vi "Call Refprop.vi"(0 "fluid name":u16(ring)=17 items=["AIR.MIX", "AMARILLO.MIX", "EKOFISK.MIX", "GLFCOAST.MIX", "HIGHCO2.MIX", "HIGHN2.MIX", "NGSAMPLE.MIX", "R401A.MIX", "R401B.MIX", "R401C.MIX", "R402A.MIX", "R402B.MIX", "R403A.MIX", "R403B.MIX", "R405A.MIX", "R406A.MIX", "R407A.MIX", "R407B.MIX", "R407C.MIX", "R407D.MIX", "R407E.MIX", "R408A.MIX", "R409A.MIX", "R409B.MIX", "R410A.PPF", "R410B.MIX", "R411A.MIX", "R411B.MIX", "R412A.MIX", "R413A.MIX", "R414B.MIX", "R415A.MIX", "R415B.MIX", "R416A.MIX", "R417A.MIX", "R417B.MIX", "R417C.MIX", "R418A.MIX", "R419A.MIX", "R419B.MIX", "R420A.MIX", "R421A.MIX", "R421B.MIX", "R422A.MIX", "R422B.MIX", "R422C.MIX", "R422D.MIX", "R423A.MIX", "R424A.MIX", "R425A.MIX", "R426A.MIX", "R427A.MIX", "R428A.MIX", "R429A.MIX", "R430A.MIX", "R431A.MIX", "R432A.MIX", "R433A.MIX", "R433B.MIX", "R433C.MIX", "R434A.MIX", "R435A.MIX", "R436A.MIX", "R436B.MIX", "R437A.MIX", "R438A.MIX", "R439A.MIX", "R440A.MIX", "R441A.MIX", "R442A.MIX", "R443A.MIX", "R444A.MIX", "R444B.MIX", "R445A.MIX", "R446A.MIX", "R447A.MIX", "R448A.MIX", "R449A.MIX", "R449B.MIX", "R450A.MIX", "R451A.MIX", "R451B.MIX", "R452A.MIX", "R452B.MIX", "R452C.MIX", "R453A.MIX", "R454A.MIX", "R454B.MIX", "R454C.MIX", "R455A.MIX", "R456A.MIX", "R457A.MIX", "R459A.MIX", "R459B.MIX", "R460A.MIX", "R460B.MIX", "R500.MIX", "R501.MIX", "R502.MIX", "R503.MIX", "R504.MIX", "R507A.MIX", "R508A.MIX", "R508B.MIX", "R509A.MIX", "R510A.MIX", "R511A.MIX", "R512A.MIX", "R513A.MIX", "R513B.MIX", "R515A.MIX", "ammonia.fld", "butane.fld", "ethane.fld", "propane.fld", "R11.fld", "R113.fld", "R114.fld", "R115.fld", "R116.fld", "R12.fld", "R123.fld", "R124.fld", "R125.fld", "R13.fld", "R134a.fld", "R14.fld", "R141b.fld", "R142b.fld", "R143a.fld", "R152a.fld", "R161.fld", "R21.fld", "R218.fld", "R22.fld", "R227ea.fld", "R23.fld", "R236ea.fld", "R236fa.fld", "R245ca.fld", "R245fa.fld", "R32.fld", "R41.fld", "R1216.fld", "RC318.fld", "water.fld", "1butene.fld", "acetone.fld", "argon.fld", "benzene.fld", "c1cc6.fld", "c2butene.fld", "c3cc6.fld", "c4f10.fld", "c5f12.fld", "c11.fld", "c12.fld", "cf3i.fld", "CO.fld", "CO2.fld", "COS.fld", "cyclohex.fld", "cyclopen.fld", "cyclopro.fld", "D2.fld", "D2O.fld", "D4.fld", "D5.fld", "D6.fld", "decane.fld", "dee.fld", "dmc.fld", "dme.fld", "ebenzene.fld", "ethanol.fld", "ethylene.fld", "flourine.fld", "H2S.fld", "HCl.fld", "helium.fld", "heptane.fld", "hexane.fld", "hydrogen.fld", "ibutene.fld", "ihexane.fld", "ioctane.fld", "ipentane.fld", "isobutan.fld", "krypton.fld", "MD2M.fld", "MD3M.fld", "MD4M.fld", "MDM.fld", "methane.fld", "methanol.fld", "mlinolea.fld", "mlinolen.fld", "MM.fld", "moleate.fld", "mpalmita.fld", "mstearat.fld", "mxylene.fld", "N2O.fld", "neon.fld", "neopentn.fld", "NF3.fld", "nitrogen.fld", "nonane.fld", "novec649.fld", "octane.fld", "orthohyd.fld", "oxygen.fld", "parahyd.fld", "pentane.fld", "propylen.fld", "propyne.fld", "pxylene.fld", "R365MFC.fld", "R1233zd.fld", "R1234yf.fld", "R1234ze.fld", "RE143a.fld", "RE245cb2.fld", "RE245fa2.fld", "RE347mcc.fld", "sf6.fld", "SO2.fld", "T2butene.fld", "xenon.fld"], 1 "units":enum16{"SI", "IP"}(ring), 5 "InpCode":T1(ring)=enum."TP", 9 "output_1":dbl=40.0, 11 "output_2":dbl=632.0) -> (4 "data":string[][](table)=[["0", "T", "40.917420"], ["1", "P", "632.917420"], ["2", "H", "466.332574"], ["3", "S", "2.054657"], ["4", "DV", "18.926081"], ["5", "DL", "18.926081"], ["6", "E", "432.891028"], ["7", "CV", "0.758226"], ["8", "CP", "0.924261"], ["9", "W", "194.299169"], ["10", "Q", "998.000000"]], 6 "Component Molar Fractions":dbl[](array[numeric]), 8 "Critical temperature (K)":dbl, 10 "Molecular Weight":dbl=72.58534253397343 format="%#_11g", 15 "Critical Pressure (kPa)":dbl)   [LabVIEW 2017]
panel:
  out "Components":i32=2
  out "refprop_main_directory":string="D:\\ni files\\refproplv\\cll_refprop_dll_on_lv"
  out "xmlout":string="<Array>\r\n<Name></Name>\r\n<Dimsize>39</Dimsize>\r\n<Dimsize>2</Dimsize>\r\n<String>\r\n<Name>String</Name>\r\n<Val>ammonia</Val>\r\n</String>\r\n<String>\r\n<Name>String</Name>\r\n<Val>ammonia</Val>\r\n</String>\r\n<String>\r\n<Name>String</Name>\r\n<Val>argon</Val>\r\n</String>\r\n<String>\r\n<Name>String</Name>\r\n<Val>argon</Val>\r\n</String>\r\n<String>\r\n<Name>String</Name>\r\n<Val>butane</Val>\r\n</String>\r\n<String>\r\n<Name>String</Name>\r\n<Val>n-butane</Val>\r\n</String>\r\n<String>\r\n<Name>String</Name>\r\n<Val>carbon dioxide</Val>\r\n</String>\r\n<String>\r\n<Name>String</Name>\r\n<Val>carbon dioxide</Val>\r\n</String>\r\n<String>\r\n<Name>String</Name>\r\n<Val>ethane</Val>\r\n</String>\r\n<String>\r\n<Name>String</Name>\r\n<Val>ethane</Val>\r\n</String>\r\n<String>\r\n<Name>String</Name>\r\n<Val>isobutane</Val>\r\n</String>\r\n<String>\r\n<Name>String</Name>\r\n<Val>2-methylpropane</Val>\r\n</String>\r\n<String>\r\n<Name>String</Name>\r\n<Val>methane</Val>\r\n</String>\r\n<String>\r\n<Name>String</Name>\r\n<Val>methane</Val>\r\n</String>\r\n<String>\r\n<Name>String</Name>\r\n<Val>nitrogen</Val>\r\n</String>\r\n<String>\r\n<Name>String</Name>\r\n<Val>nitrogen</Val>\r\n</String>\r\n<String>\r\n<Name>String</Name>\r\n<Val>oxygen</Val>\r\n</String>\r\n<String>\r\n<Name>String</Name>\r\n<Val>oxygen</Val>\r\n</String>\r\n<String>\r\n<Name>String</Name>\r\n<Val>propane</Val>\r\n</String>\r\n<String>\r\n<Name>String</Name>\r\n<Val>propane</Val>\r\n</String>\r\n<String>\r\n<Name>String</Name>\r\n<Val>propylene</Val>\r\n</String>\r\n<String>\r\n<Name>String</Name>\r\n<Val>propene</Val>\r\n</String>\r\n<String>\r\n<Name>String</Name>\r\n<Val>R11</Val>\r\n</String>\r\n<String>\r\n<Name>String</Name>\r\n<Val>trichlorofluoromethane</Val>\r\n</String>\r\n<String>\r\n<Name>String</Name>\r\n<Val>R113</Val>\r\n</String>\r\n<String>\r\n<Name>String</Name>\r\n<Val>1,1,2-trichloro-1,2,2-trifluoroethane</Val>\r\n</String>\r\n<String>\r\n<Name>String</Name>\r\n<Val>R114</Val>\r\n</String>\r\n<String>\r\n<Name>String</Name>\r\n<Val>1,2-dichloro-1,1,2,2-tetrafluoroethane</Val>\r\n</String>\r\n<String>\r\n<Name>String</Name>\r\n<Val>R115</Val>\r\n</String>\r\n<String>\r\n<Name>String</Name>\r\n<Val>chloropentafluoroethane</Val>\r\n</String>\r\n<String>\r\n<Name>String</Name>\r\n<Val>R116</Val>\r\n</String>\r\n<String>\r\n<Name>String</Name>\r\n<Val>hexafluoroethane</Val>\r\n</String>\r\n<String>\r\n<Name>String</Name>\r\n<Val>R12</Val>\r\n</String>\r\n<String>\r\n<Name>String</Name>\r\n<Val>dichlorodifluoromethane</Val>\r\n</String>\r\n<String>\r\n<Name>String</Name>\r\n<Val>R123</Val>\r\n</String>\r\n<String>\r\n<Name>String</Name>\r\n<Val>2,2-dichloro-1,1,1-trifluoroethane</Val>\r\n</String>\r\n<String>\r\n<Name>String</Name>\r\n<Val>R124</Val>\r\n</String>\r\n<String>\r\n<Name>String</Name>\r\n<Val>1-chloro-1,2,2,2-tetrafluoroethane</Val>\r\n</String>\r\n<String>\r\n<Name>String</Name>\r\n<Val>R125</Val>\r\n</String>\r\n<String>\r\n<Name>String</Name>\r\n<Val>pentafluoroethane</Val>\r\n</String>\r\n<String>\r\n<Name>String</Name>\r\n<Val>R13</Val>\r\n</String>\r\n<String>\r\n<Name>String</Name>\r\n<Val>chlorotrifluoromethane</Val>\r\n</String>\r\n<String>\r\n<Name>String</Name>\r\n<Val>R134a</Val>\r\n</String>\r\n<String>\r\n<Name>String</Name>\r\n<Val>1,1,1,2-tetrafluoroethane</Val>\r\n</String>\r\n<String>\r\n<Name>String</Name>\r\n<Val>R14</Val>\r\n</String>\r\n<String>\r\n<Name>String</Name>\r\n<Val>tetrafluoromethane</Val>\r\n</String>\r\n<String>\r\n<Name>String</Name>\r\n<Val>R141b</Val>\r\n</String>\r\n<String>\r\n<Name>String</Name>\r\n<Val>1,1-dichloro-1-fluoroethane</Val>\r\n</String>\r\n<String>\r\n<Name>String</Name>\r\n<Val>R142b</Val>\r\n</String>\r\n<String>\r\n<Name>String</Name>\r\n<Val>1-chloro-1,1-difluoroethane</Val>\r\n</String>\r\n<String>\r\n<Name>String</Name>\r\n<Val>R143a</Val>\r\n</String>\r\n<String>\r\n<Name>String</Name>\r\n<Val>1,1,1-trifluoroethane</Val>\r\n</String>\r\n<String>\r\n<Name>String</Name>\r\n<Val>R152a</Val>\r\n</String>\r\n<String>\r\n<Name>String</Name>\r\n<Val>1,1-difluoroethane</Val>\r\n</String>\r\n<String>\r\n<Name>String</Name>\r\n<Val>R218</Val>\r\n</String>\r\n<String>\r\n<Name>String</Name>\r\n<Val>octafluoropropane</Val>\r\n</String>\r\n<String>\r\n<Name>String</Name>\r\n<Val>R22</Val>\r\n</String>\r\n<String>\r\n<Name>String</Name>\r\n<Val>chlorodifluoromethane</Val>\r\n</String>\r\n<String>\r\n<Name>String</Name>\r\n<Val>R227ea</Val>\r\n</String>\r\n<String>\r\n<Name>String</Name>\r\n<Val>1,1,1,2,3,3,3-heptafluoropropane</Val>\r\n</String>\r\n<String>\r\n<Name>String</Name>\r\n<Val>R23</Val>\r\n</String>\r\n<String>\r\n<Name>String</Name>\r\n<Val>trifluoromethane</Val>\r\n</String>\r\n<String>\r\n<Name>String</Name>\r\n<Val>R236ea</Val>\r\n</String>\r\n<String>\r\n<Name>String</Name>\r\n<Val>1,1,1,2,3,3-hexafluoropropane</Val>\r\n</String>\r\n<String>\r\n<Name>String</Name>\r\n<Val>R236fa</Val>\r\n</String>\r\n<String>\r\n<Name>String</Name>\r\n<Val>1,1,1,3,3,3-hexafluoropropane</Val>\r\n</String>\r\n<String>\r\n<Name>String</Name>\r\n<Val>R245ca</Val>\r\n</String>\r\n<String>\r\n<Name>String</Name>\r\n<Val>1,1,2,2,3-pentafluoropropane</Val>\r\n</String>\r\n<String>\r\n<Name>String</Name>\r\n<Val>R245fa</Val>\r\n</String>\r\n<String>\r\n<Name>String</Name>\r\n<Val>1,1,1,3,3-pentafluoropropane</Val>\r\n</String>\r\n<String>\r\n<Name>String</Name>\r\n<Val>R32</Val>\r\n</String>\r\n<String>\r\n<Name>String</Name>\r\n<Val>difluoromethane</Val>\r\n</String>\r\n<String>\r\n<Name>String</Name>\r\n<Val>R41</Val>\r\n</String>\r\n<String>\r\n<Name>String</Name>\r\n<Val>fluoromethane</Val>\r\n</String>\r\n<String>\r\n<Name>String</Name>\r\n<Val>RC318</Val>\r\n</String>\r\n<String>\r\n<Name>String</Name>\r\n<Val>octafluorocyclobutane</Val>\r\n</String>\r\n<String>\r\n<Name>String</Name>\r\n<Val>water</Val>\r\n</String>\r\n<String>\r\n<Name>String</Name>\r\n<Val>water</Val>\r\n</String>\r\n</Array>\r\n"
  out "xmlout 2":string="<Array>\r\n<Name></Name>\r\n<Dimsize>35</Dimsize>\r\n<Dimsize>2</Dimsize>\r\n<String>\r\n<Name>String</Name>\r\n<Val>Air</Val>\r\n</String>\r\n<String>\r\n<Name>String</Name>\r\n<Val>NITROGEN (78.12%), ARGON (0.92%), OXYGEN (20.96%)</Val>\r\n</String>\r\n<String>\r\n<Name>String</Name>\r\n<Val>R401A</Val>\r\n</String>\r\n<String>\r\n<Name>String</Name>\r\n<Val>R22 (57.89%), R152A (18.59%), R124 (23.53%)</Val>\r\n</String>\r\n<String>\r\n<Name>String</Name>\r\n<Val>R401B</Val>\r\n</String>\r\n<String>\r\n<Name>String</Name>\r\n<Val>R22 (65.49%), R152A (15.46%), R124 (19.05%)</Val>\r\n</String>\r\n<String>\r\n<Name>String</Name>\r\n<Val>R401C</Val>\r\n</String>\r\n<String>\r\n<Name>String</Name>\r\n<Val>R22 (38.56%), R152A (22.94%), R124 (38.50%)</Val>\r\n</String>\r\n<String>\r\n<Name>String</Name>\r\n<Val>R402A</Val>\r\n</String>\r\n<String>\r\n<Name>String</Name>\r\n<Val>R125 (50.77%), PROPANE (4.61%), R22 (44.63%)</Val>\r\n</String>\r\n<String>\r\n<Name>String</Name>\r\n<Val>R402B</Val>\r\n</String>\r\n<String>\r\n<Name>String</Name>\r\n<Val>R125 (29.99%), PROPANE (4.30%), R22 (65.72%)</Val>\r\n</String>\r\n<String>\r\n<Name>String</Name>\r\n<Val>R403A</Val>\r\n</String>\r\n<String>\r\n<Name>String</Name>\r\n<Val>PROPANE (10.43%), R22 (79.79%), R218 (9.78%)</Val>\r\n</String>\r\n<String>\r\n<Name>String</Name>\r\n<Val>R403B</Val>\r\n</String>\r\n<String>\r\n<Name>String</Name>\r\n<Val>PROPANE (11.71%), R22 (66.87%), R218 (21.42%)</Val>\r\n</String>\r\n<String>\r\n<Name>String</Name>\r\n<Val>R404A</Val>\r\n</String>\r\n<String>\r\n<Name>String</Name>\r\n<Val>R125 (35.78%), R143A (60.39%), R134A (3.83%)</Val>\r\n</String>\r\n<String>\r\n<Name>String</Name>\r\n<Val>R405A</Val>\r\n</String>\r\n<String>\r\n<Name>String</Name>\r\n<Val>R22 (58.24%), R152A (11.86%), R142B (6.12%), RC318 (23.78%)</Val>\r\n</String>\r\n<String>\r\n<Name>String</Name>\r\n<Val>R406A</Val>\r\n</String>\r\n<String>\r\n<Name>String</Name>\r\n<Val>R22 (57.16%), ISOBUTAN (6.18%), R142B (36.66%)</Val>\r\n</String>\r\n<String>\r\n<Name>String</Name>\r\n<Val>R407A</Val>\r\n</String>\r\n<String>\r\n<Name>String</Name>\r\n<Val>R32 (34.64%), R125 (30.03%), R134A (35.33%)</Val>\r\n</String>\r\n<String>\r\n<Name>String</Name>\r\n<Val>R407B</Val>\r\n</String>\r\n<String>\r\n<Name>String</Name>\r\n<Val>R32 (19.79%), R125 (60.04%), R134A (20.18%)</Val>\r\n</String>\r\n<String>\r\n<Name>String</Name>\r\n<Val>R407C</Val>\r\n</String>\r\n<String>\r\n<Name>String</Name>\r\n<Val>R32 (38.11%), R125 (17.96%), R134A (43.93%)</Val>\r\n</String>\r\n<String>\r\n<Name>String</Name>\r\n<Val>R407D</Val>\r\n</String>\r\n<String>\r\n<Name>String</Name>\r\n<Val>R32 (26.23%), R125 (11.37%), R134A (62.41%)</Val>\r\n</String>\r\n<String>\r\n<Name>String</Name>\r\n<Val>R407E</Val>\r\n</String>\r\n<String>\r\n<Name>String</Name>\r\n<Val>R32 (40.26%), R125 (10.47%), R134A (49.27%)</Val>\r\n</String>\r\n<String>\r\n<Name>String</Name>\r\n<Val>R408A</Val>\r\n</String>\r\n<String>\r\n<Name>String</Name>\r\n<Val>R125 (5.07%), R143A (47.63%), R22 (47.30%)</Val>\r\n</String>\r\n<String>\r\n<Name>String</Name>\r\n<Val>R409A</Val>\r\n</String>\r\n<String>\r\n<Name>String</Name>\r\n<Val>R22 (67.61%), R124 (17.85%), R142B (14.54%)</Val>\r\n</String>\r\n<String>\r\n<Name>String</Name>\r\n<Val>R409B</Val>\r\n</String>\r\n<String>\r\n<Name>String</Name>\r\n<Val>R22 (72.67%), R124 (17.71%), R142B (9.62%)</Val>\r\n</String>\r\n<String>\r\n<Name>String</Name>\r\n<Val>R410A</Val>\r\n</String>\r\n<String>\r\n<Name>String</Name>\r\n<Val>R32 (69.76%), R125 (30.24%)</Val>\r\n</String>\r\n<String>\r\n<Name>String</Name>\r\n<Val>R410B</Val>\r\n</String>\r\n<String>\r\n<Name>String</Name>\r\n<Val>R32 (65.37%), R125 (34.63%)</Val>\r\n</String>\r\n<String>\r\n<Name>String</Name>\r\n<Val>R411A</Val>\r\n</String>\r\n<String>\r\n<Name>String</Name>\r\n<Val>PROPYLEN (2.94%), R22 (83.35%), R152A (13.72%)</Val>\r\n</String>\r\n<String>\r\n<Name>String</Name>\r\n<Val>R411B</Val>\r\n</String>\r\n<String>\r\n<Name>String</Name>\r\n<Val>PROPYLEN (5.92%), R22 (90.30%), R152A (3.77%)</Val>\r\n</String>\r\n<String>\r\n<Name>String</Name>\r\n<Val>R412A</Val>\r\n</String>\r\n<String>\r\n<Name>String</Name>\r\n<Val>R22 (74.62%), R218 (2.45%), R142B (22.93%)</Val>\r\n</String>\r\n<String>\r\n<Name>String</Name>\r\n<Val>R413A</Val>\r\n</String>\r\n<String>\r\n<Name>String</Name>\r\n<Val>R218 (4.98%), R134A (89.66%), ISOBUTAN (5.37%)</Val>\r\n</String>\r\n<String>\r\n<Name>String</Name>\r\n<Val>R414B</Val>\r\n</String>\r\n<String>\r\n<Name>String</Name>\r\n<Val>R22 (58.74%), R124 (29.03%), ISOBUTAN (2.62%), R142B (9.60%)</Val>\r\n</String>\r\n<String>\r\n<Name>String</Name>\r\n<Val>R500</Val>\r\n</String>\r\n<String>\r\n<Name>String</Name>\r\n<Val>R12 (60.61%), R152A (39.39%)</Val>\r\n</String>\r\n<String>\r\n<Name>String</Name>\r\n<Val>R501</Val>\r\n</String>\r\n<String>\r\n<Name>String</Name>\r\n<Val>R22 (80.75%), R12 (19.25%)</Val>\r\n</String>\r\n<String>\r\n<Name>String</Name>\r\n<Val>R502</Val>\r\n</String>\r\n<String>\r\n<Name>String</Name>\r\n<Val>R22 (63.00%), R115 (37.00%)</Val>\r\n</String>\r\n<String>\r\n<Name>String</Name>\r\n<Val>R503</Val>\r\n</String>\r\n<String>\r\n<Name>String</Name>\r\n<Val>R23 (49.97%), R13 (50.03%)</Val>\r\n</String>\r\n<String>\r\n<Name>String</Name>\r\n<Val>R504</Val>\r\n</String>\r\n<String>\r\n<Name>String</Name>\r\n<Val>R32 (73.42%), R115 (26.58%)</Val>\r\n</String>\r\n<String>\r\n<Name>String</Name>\r\n<Val>R507A</Val>\r\n</String>\r\n<String>\r\n<Name>String</Name>\r\n<Val>R125 (41.18%), R143A (58.82%)</Val>\r\n</String>\r\n<String>\r\n<Name>String</Name>\r\n<Val>R508A</Val>\r\n</String>\r\n<String>\r\n<Name>String</Name>\r\n<Val>R23 (55.76%), R116 (44.24%)</Val>\r\n</String>\r\n<String>\r\n<Name>String</Name>\r\n<Val>R508B</Val>\r\n</String>\r\n<String>\r\n<Name>String</Name>\r\n<Val>R23 (62.67%), R116 (37.33%)</Val>\r\n</String>\r\n<String>\r\n<Name>String</Name>\r\n<Val>R509A</Val>\r\n</String>\r\n<String>\r\n<Name>String</Name>\r\n<Val>R22 (63.08%), R218 (36.92%)</Val>\r\n</String>\r\n</Array>\r\n"
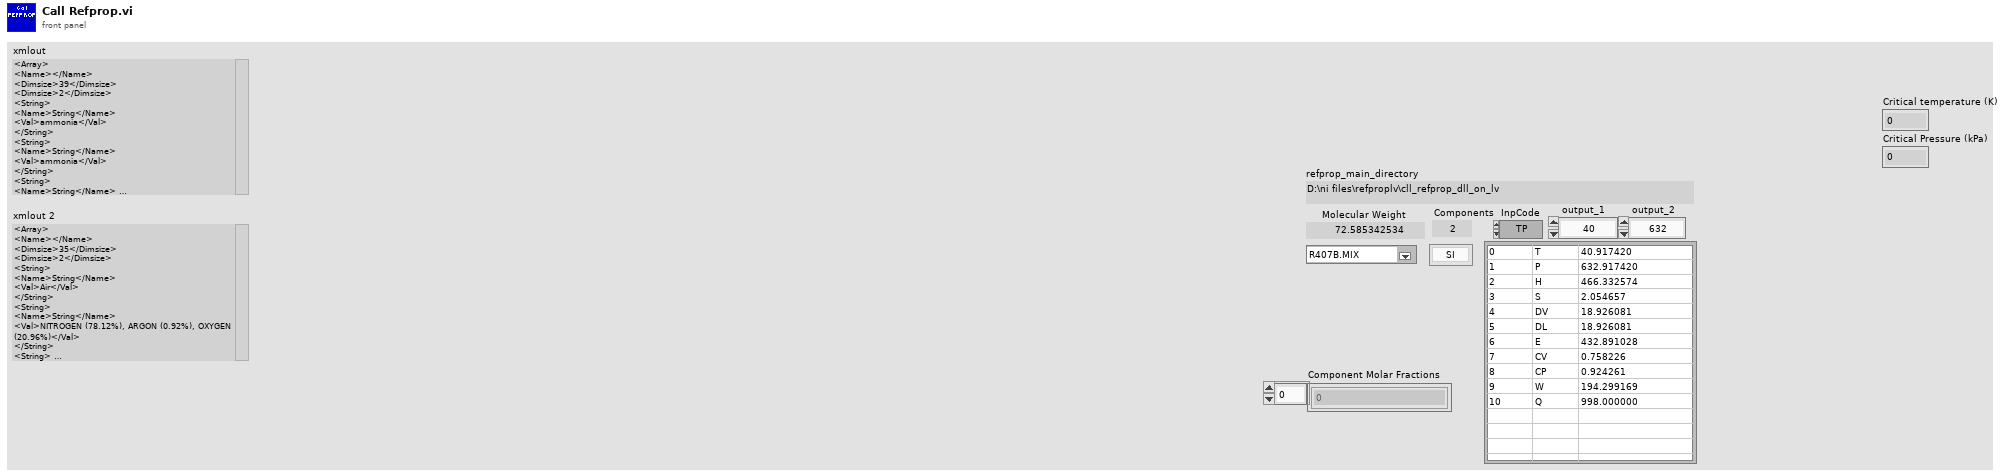
[diagram p1: front panel]
types:
  T1 = enum16{"0", "PS", "HS", "T", "P", "TP", "TH", "TS", "PH", "PQ", "TQ"}
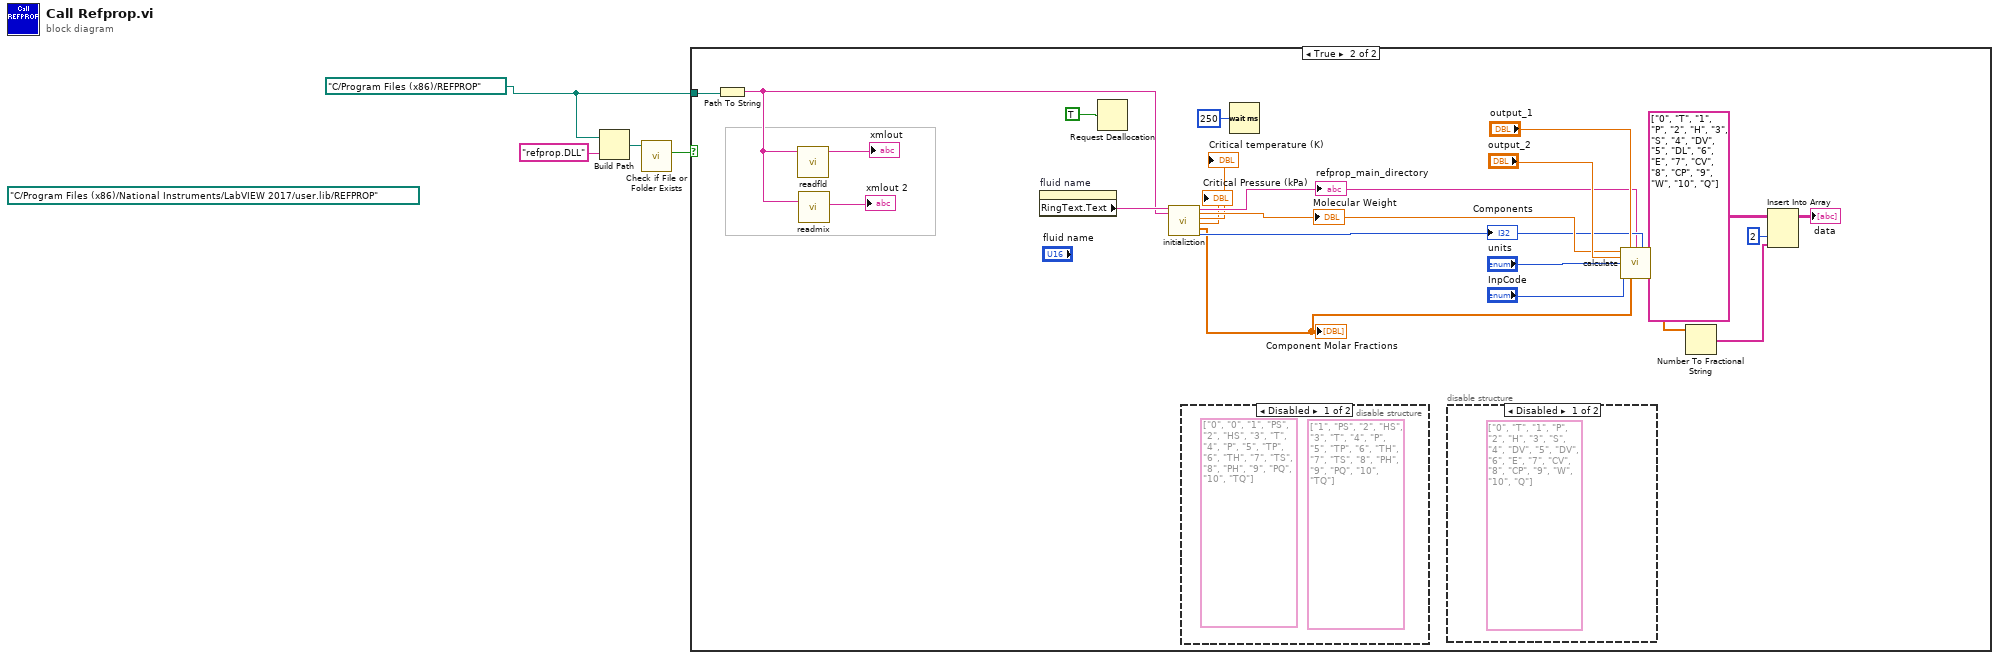
[diagram p0: block diagram]
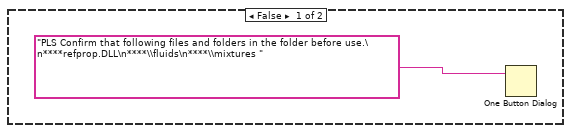
[diagram p2: hidden frame]
diagram:
  (unwired) path "C:/Program Files (x86)/National Instruments/LabVIEW 2017/user.lib/REFPROP" ("start path")
  w1 = path "C:/Program Files (x86)/REFPROP" ("start path")
  n1 = Build Path(base path=w1, name or relative path="refprop.DLL" ("名称或相对路径")) -> (appended path=w3:path)
  n2 = call <vilib>:"Check if File or Folder Exists.vi"("path"=w3) -> ("file or folder exists?"=w2:bool)  [unwired: 8 in, 2 out]
  n3 = case shown="True" w2 {
    tunnel: w1 -> [_ w25]
    frame False {
      n4 = One Button Dialog(message="PLS Confirm that following files and folders in the folder before use.\n****refprop.DLL\n****\\fluids\n****\\mixtures " ("消息")) -> ()  [unwired: 1 in, 1 out]
    }
    frame True {
      n5 = Path To String(path=w25) -> (string=w9:string)
      n6 = call "readfld.vi"("path"=w9) -> ("xmlout"=→"xmlout":string)  [unwired: 10 in]
      n7 = call "readmix.vi"("path"=w9) -> ("xmlout"=→"xmlout 2":string)  [unwired: 10 in]
      n8 = property on="fluid name" class="Ring (strict)"() -> ("RingText.Text"=w18:string)  [unwired: 2 in, 2 out]
      n9 = Request Deallocation(TRUE ("标志")) -> ()
      n10 = call "initializtion.vi"("Fluidofinterest"=w18, "path"=w9) -> ("refprop _main_directory"=w11:string, "Molecular Weight"=w15:dbl, "Critical temperature (K)"=→"Critical temperature (K)":dbl, "Critical Pressure (kPa)"=→"Critical Pressure (kPa)":dbl, "Component Molar Fractions"=w8:dbl[], "Components"=w12:i32)  [unwired: 12 in]
      "refprop_main_directory" <- w11
      "Molecular Weight" <- w15
      "Component Molar Fractions" <- w8
      "Components" <- w12
      n11 = disable-structure shown="Disabled" {
        frame Disabled {
          (unwired) string[][] [["1", "PS"], ["2", "HS"], ["3", "T"], ["4", "P"], ["5", "TP"], ["6", "TH"], ["7", "TS"], ["8", "PH"], ["9", "PQ"], ["10", "TQ"]]
          (unwired) string[][] [["0", "0"], ["1", "PS"], ["2", "HS"], ["3", "T"], ["4", "P"], ["5", "TP"], ["6", "TH"], ["7", "TS"], ["8", "PH"], ["9", "PQ"], ["10", "TQ"]]
        }
        frame Enabled {
        }
      }
      n12 = Wait (ms)(milliseconds to wait=u32 250 ("等待时间（毫秒）")) -> ()  [unwired: 1 out]
      n13 = disable-structure shown="Disabled" {
        frame Disabled {
          (unwired) string[][] [["0", "T"], ["1", "P"], ["2", "H"], ["3", "S"], ["4", "DV"], ["5", "DV"], ["6", "E"], ["7", "CV"], ["8", "CP"], ["9", "W"], ["10", "Q"]]
        }
        frame Enabled {
        }
      }
      n14 = call "calculate.vi"("wm"=w15, "input_1"="output_1", "RefpropDirectory"=w11, "n"=w12, "input_2"="output_2", "units"="units", "InpCode"="InpCode", "x"=w8) -> ("dataout"=w10:dbl[])  [unwired: 5 in, 2 out]
      n15 = Number To Fractional String(number=w10) -> (F-format string=w22:string[])  [unwired: 3 in]
      n16 = Insert Into Array(array=string[][] [["0", "T"], ["1", "P"], ["2", "H"], ["3", "S"], ["4", "DV"], ["5", "DL"], ["6", "E"], ["7", "CV"], ["8", "CP"], ["9", "W"], ["10", "Q"]] ("数组"), index (col)=2 ("禁用的索引 (列)"), new element=w22) -> (→"data":string[][])  [unwired: 1 in]
    }
  }
